vi "Load Config File (SubVI).vi"() -> (0 "sortie d'erreur":errorcluster, 2 "Type .EXE":bool, 3 "*(type *) &x":refnum<k21>)   [LabVIEW 2017]
doc: "by Tanguy BOULARD"
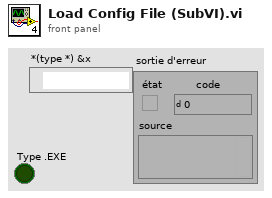
[diagram p1: front panel]
types:
  T1 = enum32{"invalid app kind", "Development System", "Run Time System", "Student Edition", "Embedded LabVIEW", "Evaluation", "Custom"}
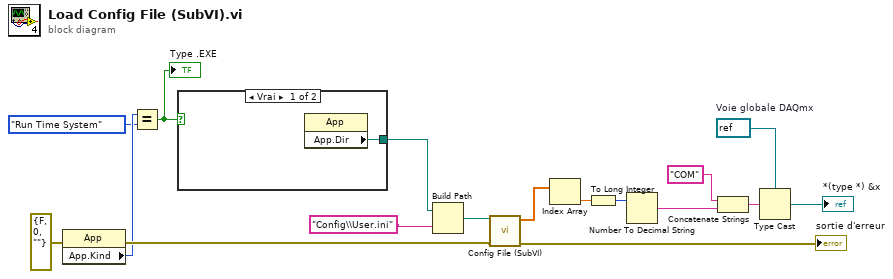
[diagram p0: block diagram]
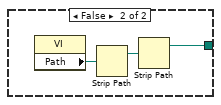
[diagram p2: hidden frame]
diagram:
  w2 = refnum<k21> refnum  # Voie globale DAQmx
  n1 = property class="App"(error in=errorcluster {"status"=FALSE, "code"=0, "source"=""} ("error out")) -> (error out=w11:errorcluster, "App.Kind"=w5:T1)  [unwired: 1 in, 1 out]
  n2 = Equal?(x=w5, y=T1."Run Time System" ("Application:Kind")) -> (x = y?=w8:bool)
  "Type .EXE" <- w8
  n3 = case shown="Vrai" w8 {
    tunnel: [w18 w19] -> w9
    frame True {
      n4 = property class="App"() -> ("App.Dir"=w18:path)  [unwired: 2 in, 2 out]
    }
    frame False {
      n5 = property class="VI"() -> ("Path"=w20:path)  [unwired: 2 in, 2 out]
      n6 = Strip Path(path=w20) -> (stripped path=w21:path)  [unwired: 1 out]
      n7 = Strip Path(path=w21) -> (stripped path=w19:path)  [unwired: 1 out]
    }
  }
  n8 = Build Path(base path=w9, name or relative path="Config\\User.ini" ("User_file_name")) -> (appended path=w10:path)
  n9 = call "Config File (SubVI).vi"("entrée d'erreur (pas d'erreur)"=w11, "configuration file path"=w10) -> ("sortie d'erreur"=→"sortie d'erreur":errorcluster, "User file contents"=w16:dbl[])  [unwired: 8 in]
  n10 = Index Array(array=w16) -> (element=w17:dbl)  [unwired: 1 in]
  n11 = To Long Integer(number=w17) -> (32bit integer=w13:i32)
  n12 = Number To Decimal String(number=w13) -> (decimal integer string=w14:string)  [unwired: 1 in]
  n13 = Concatenate Strings("COM" ("string"), w14) -> (w15:string)
  n14 = Type Cast(type=w2, x=w15) -> (*(type *) &x=→"*(type *) &x":refnum<k21>)
